vi "Cont Acq&Chart Samples-Int Clk-Dig Start.vi"() -> ()   [LabVIEW 2011]
doc: "I. Description:\nThis example demonstrates how to continuously acquire data (Waveform) using the DAQ device's internal clock and a digital start trigger.\n\nII. Instructions for Running:\n1. Select the physical channel to correspond to where your signal is input on the DAQ device.\n2. Enter the minimum and maximum voltage ranges.\nNote: For better accuracy try to match the input range to the expected voltage level of the measured signal.\n3. Set the sample rate of the acquisition. Also set the Samples to Read control. This will determine how many samples are read each time the while loop iterates. This also determines how many points are plotted on the chart each iteration.\nNote: The rate should be AT LEAST twice as fast as the maximum frequency component of the signal being acquired.\n4. Select the Source of the Digital Start Trigger for the acquisition.\n5. Select the edge, rising or falling, on which to trigger.\n\nIII. Block Diagram Steps:\n1. Create an analog input voltage channel.\n2. Set the rate for the sample clock. Additionally, define the sample mode to be continuous.\n3. Define the parameters for a Digital Edge Start Trigger\n4. Call the Start VI to start acquiring samples.\n5. Read the waveform data in a loop until the user hits the stop button or an error occurs.\n6. Call the Clear Task VI to clear the Task.\n7. Use the popup dialog box to display an error if any.\n\nIV. I/O Connections Overview:\nMake sure your signal input terminal matches the Physical Channel I/O control. Also, make sure your digital trigger terminal matches the Trigger Source Control. For further connection information, refer to your hardware reference manual."
uses:
  DialogType.ctl
  DAQmx Read (Analog 1D Wfm NChan NSamp).vi
  DAQmx Create Channel (AI-Voltage-Basic).vi
  DAQmx Timing (Sample Clock).vi
  DAQmx Start Trigger (Digital Edge).vi
  DAQmx Fill In Error Info.vi
panel:
  in  "Samples to Read":i32=10
  in  "Slope":i32(ring)=10280 items=["Rising"=10280, "Falling"=10171]
  in  "Trigger Source":tag="/Dev1/PFI0"
  in  "Maximum Value":dbl=10.0 format="%0.2f"
  in  "Minimum Value":dbl=-10.0 format="%0.2f"
  in  "Physical Channel":tag="Dev1/ai0"
  in  "Rate":dbl=100.0 caption="Rate (Hz)" format="%0.2f"
  in  "stop":bool
  out "Measurement":waveform(dbl)[](graph)
  # "For instructions, select Help>>Show Context Help"
  # "Channel Parameters"
  # "Timing Parameters"
  # "Trigger Parameters"
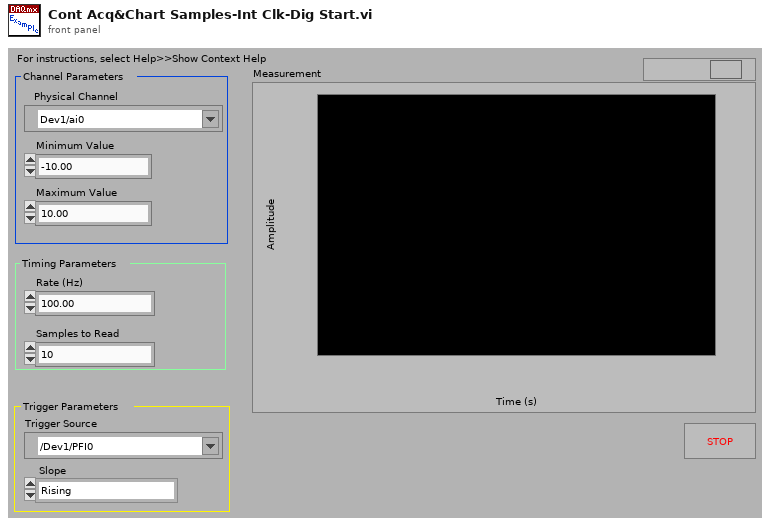
[diagram p1: front panel]
types:
  T1 = typedef "DialogType.ctl" = u16
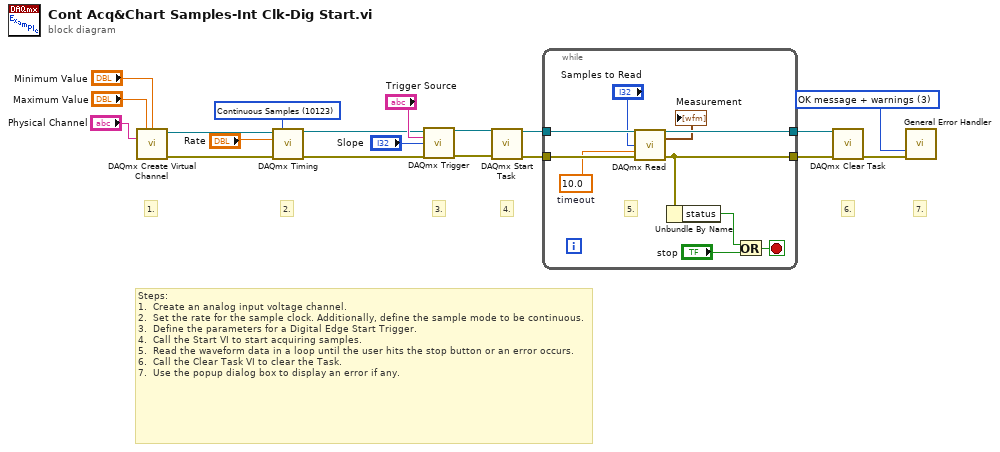
[diagram p0: block diagram]
diagram:
  w1 = T1 3 items=["no dialog", "OK message", "continue or stop message", "OK message + warnings", "continue/stop + warnings"] ("type of dialog (OK msg:1)")
  w8 = 10123 items=["Finite Samples"=10178, "Continuous Samples"=10123] ("sample mode")
  # "3."
  # "7."
  # "4."
  # "6."
  # "Steps: \n1.  Create an analog input voltage channel.\n2.  Set the rate for the sample clock. Additionally, define the sample mode to be continuous.\n3.  Define the parameters for a Digital Edge Start Trigger.\n4.  Call the Start VI to start acquiring samples.\n5.  Read the waveform data in a loop until the user hits the stop button or an error occurs.\n6.  Call the Clear Task VI to clear the Task.\n7.  Use the popup dialog box to display an error if any."
  # "2."
  # "1."
  n1 = call-poly "DAQmx Create Virtual Channel.vi"("maximum value"="Maximum Value", "minimum value"="Minimum Value", "physical channels"="Physical Channel") -> ("task out"=w12:refnum<k21>, "error out"=w17:errorcluster)  [unwired: 11 in]
  n2 = call-poly "DAQmx Timing.vi"("task/channels in"=w12, "sample mode"=w8, "rate"="Rate", "error in"=w17) -> ("task out"=w5:refnum<k21>, "error out"=w4:errorcluster)  [unwired: 10 in]
  n3 = call-poly "DAQmx Trigger.vi"("task/channels in"=w5, "source"="Trigger Source", "edge"="Slope", "error in"=w4) -> ("task out"=w2:refnum<k21>, "error out"=w3:errorcluster)  [unwired: 10 in]
  n4 = call "DAQmx Start Task.vi"("task/channels in"=w2, "error in"=w3) -> ("task out"=w11:refnum<k21>, "error out"=w16:errorcluster)  [unwired: 12 in]
  n5 = while {
    tunnel: w16 -> [w29]
    tunnel: [w25] -> w15
    tunnel: w11 -> [w24]
    tunnel: [w23] -> w10
    stop <- w28 stop-if-true
    w21 = 10.0  # timeout
    # "5."
    n6 = call-poly "DAQmx Read.vi"("task/channels in"=w24, "number of samples per channel"="Samples to Read", "timeout"=w21, "error in"=w29) -> ("task out"=w23:refnum<k21>, "data"=→"Measurement":waveform(dbl)[], "error out"=w25:errorcluster)  [unwired: 9 in]
    n7 = Unbundle By Name(w25) -> ("status"=w26:bool)
    n8 = Or(x=w26, y="stop") -> (x .or. y?=w28:bool)
  }
  n9 = call "DAQmx Clear Task.vi"("task in"=w10, "error in"=w15) -> ("error out"=w14:errorcluster)  [unwired: 13 in]
  n10 = call "General Error Handler.vi"("type of dialog (OK msg:1)"=w1, "error in (no error)"=w14) -> ()  [unwired: 9 in, 5 out]
